vi "termalImage.vi"() -> ()   [LabVIEW 2018]
doc: "This example performs writes and reads on a serial port, as directed by the user. You can press the Write and Read buttons, and change the Read Count, while the example is running.\n\nThe parameters set for the serial port must match the parameters of the connected instrument or device. In this example, the Read Count parameter specifies the number of bytes that the serial port reads. If there were more bytes at the port than the specified number, those bytes would not be read. If there were less bytes at the port than the specified number, you would receive a timeout error.\n\nThis example expands upon the flow control options for XON and XOFF, allowing the user to choose those control characters. Also, the user can enable or disable a termination character. Some devices require a termination character in order to identify the end of command strings. Some devices send a termination character to signify the end of data to be read. This example shows how you can end the Read operation once a termination character is detected in the buffer and/or append a termination character at the end of the Write data."
uses:
  <vilib>/Instr/_visa.llb/VISA Configure Serial Port (Instr).vi
panel:
  out "waiting":string
  out "Intensity Graph":dbl[][](graph)
  out "frameData":string
  in  "Stop":bool
  in  "VISA resource name":refnum<visa-resource-name>="COM6"
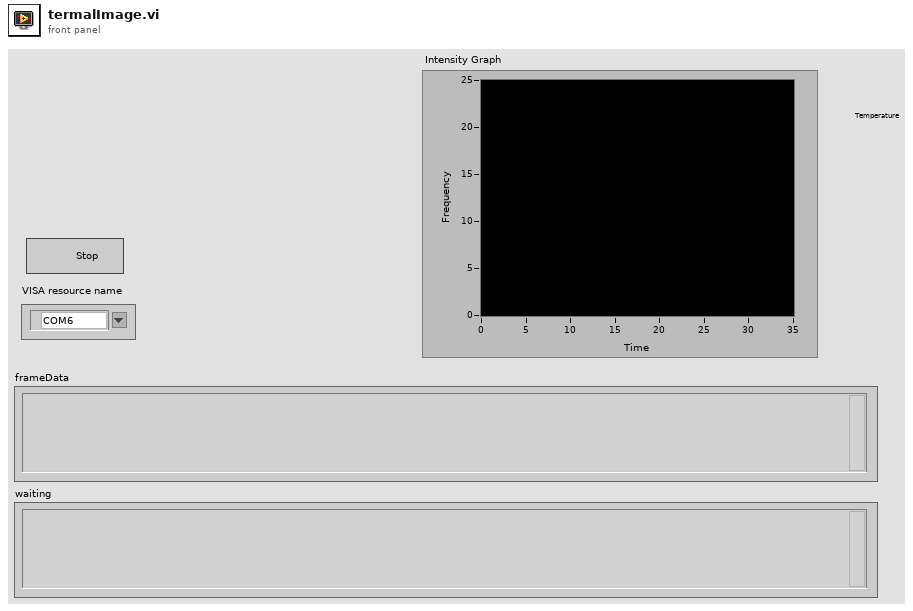
[diagram p1: front panel]
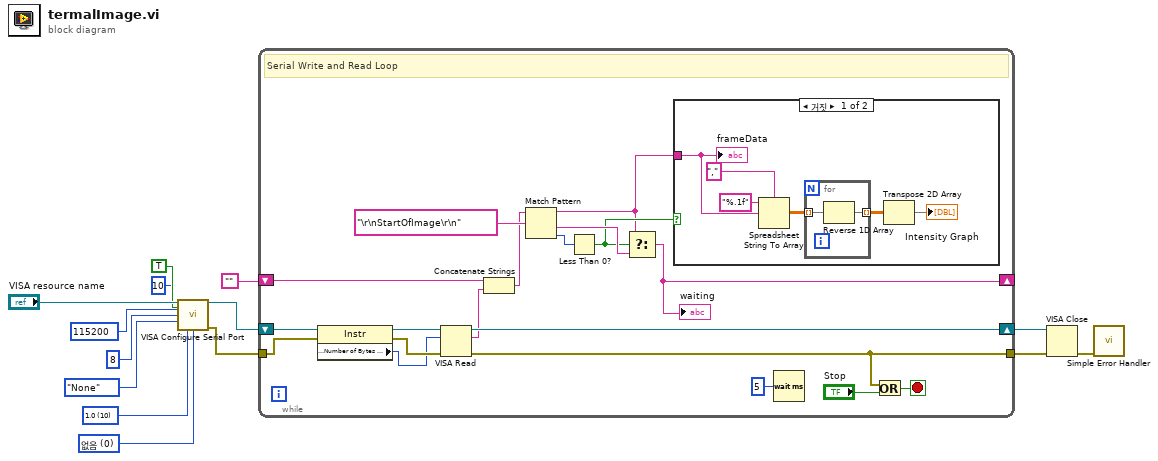
[diagram p0: block diagram]
diagram:
  w1 = u16 0 items=["없음", "XON/XOFF", "RTS/CTS", "XON/XOFF & RTS/CTS", "DTR/DSR", "XON/XOFF & DTR/DSR"] ("flow control (0:none)")
  w2 = u16 10 items=["1.0"=10, "1.5"=15, "2.0"=20] ("stop bits (10: 1 bit)")
  n1 = call-poly "VISA Configure Serial Port"("VISA resource name"="VISA resource name", "termination char\n(0xA = '\\n' = LF)"=u8 10 ("Termination Character"), "Enable Termination\nChar (T)"=TRUE ("End Read on Termination Character?"), "baud rate (9600)"=u32 115200, "data bits (8)"=u16 8, "parity (0:none)"=enum16{"None", "Odd", "Even", "Mark", "Space"}."None", "stop bits (10: 1 bit)"=w2, "flow control (0:none)"=w1) -> ("VISA resource name out"=w8:refnum<visa-resource-name>, "error out"=w7:errorcluster)  [unwired: 2 in, 4 out]
  n2 = while {
    shift-right: [w28] -> w10
    shift-left: w8 -> [w30]
    tunnel: w7 -> [w26]
    tunnel: [w22] -> w11
    shift-right: [w15] -> _
    shift-left: "" -> [w24]
    stop <- w32 stop-if-true
    # "Serial Write and Read Loop"
    n3 = property class="Instr"(reference=w30, error in=w26) -> (reference out=w29:refnum<visa-resource-name>, error out=w27:errorcluster, "Serial Settings:Number of Bytes at Serial Port"=w25:u32)
    n4 = VISA Read(VISA resource name=w29, byte count=w25, error in (no error)=w27) -> (VISA resource name out=w28:refnum<visa-resource-name>, read buffer=w23:string, error out=w22:errorcluster)  [unwired: 1 out]
    n5 = Concatenate Strings(w24, w23) -> (w20:string)
    n6 = Match Pattern(string=w20, regular expression="\r\nStartOfImage\r\n") -> (before substring=w16:string, after substring=w18:string, offset past match=w19:i32)  [unwired: 1 in, 1 out]
    n7 = Less Than 0?(x=w19) -> (x < 0?=w17:bool)
    n8 = Select(t=w16, s=w17, f=w18) -> (s? t:f=w15:string)
    "waiting" <- w15
    n9 = case shown="거짓" w17 {
      tunnel: w16 -> [w38 _]
      frame False {
        n10 = Spreadsheet String To Array(delimiter (Tab)=",", format string="%.1f", spreadsheet string=w38) -> (array=w36:dbl[][])  [unwired: 1 in]
        n11 = for {
          tunnel: w36 -> [w41] mode=indexing
          tunnel: [w40] -> w35 mode=indexing
          n12 = Reverse 1D Array(array=w41) -> (reversed array=w40:dbl[])
        }
        n13 = Transpose 2D Array(2D array=w35) -> (transposed array=→"Intensity Graph":dbl[][])
        "frameData" <- w38
      }
      frame True {
      }
    }
    n14 = Wait (ms)(milliseconds to wait=u32 5) -> ()  [unwired: 1 out]
    n15 = Or(x=w22, y="Stop") -> (x .or. y?=w32:bool)
  }
  n16 = VISA Close(VISA resource name=w10, error in (no error)=w11) -> (error out=w12:errorcluster)
  n17 = call <vilib>:"Simple Error Handler.vi"("error in (no error)"=w12) -> ()  [unwired: 1 in, 8 out]
